vi "Write cData.vi"(8 "error in":errorcluster, 10 "Data":string, 11 "hSession In":T1) -> (0 "error out":errorcluster, 3 "hSession Out":T1)   [LabVIEW 2019, in "Text Device Session.lvclass"]
uses:
  Text Device Session.lvclass
  <vilib>/MSR Consulting, LLC/General Reuse/Session APIs/_Session Fwk/Typedefs/Session Handle.ctl
  <vilib>/MSR Consulting, LLC/General Reuse/Session APIs/_Session Fwk/Session - Root.lvclass
  C:/Program Files (x86)/National Instruments/LabVIEW 2019/vi.lib/MSR Consulting, LLC/General Reuse/Session APIs/_Session Fwk/Session - Root.lvclass
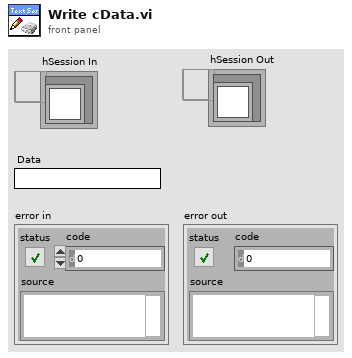
[diagram p1: front panel]
types:
  T1 = typedef "Session - Root.lvclass/Session Handle.ctl" = refnum<data-value>
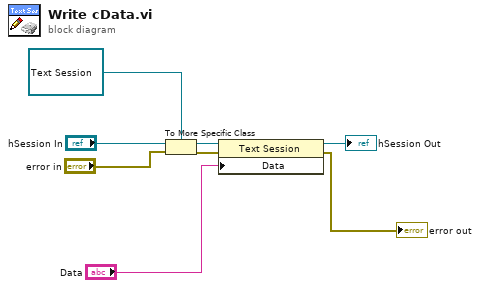
[diagram p0: block diagram]
diagram:
  n1 = To More Specific Class(target class=refnum<data-value> refnum ("hSession In"), reference="hSession In", error in="error in") -> (specific class reference=w6:refnum<data-value>, error out=w5:errorcluster)
  n2 = property class="Text Session"(reference=w6, error in=w5, "Data"="Data") -> (reference out=→"hSession Out":refnum<data-value>, error out=→"error out":errorcluster)
